vi "MFP assistant - Litho object manager.vi"(11 "Cluster":T1={"Objects to enable"=["r3", "p0", "p3"], "Only enable items in array ?"=FALSE, "All objects"=enum."Do nothing", "Funnel"=enum."Do nothing", "Path"=enum."Do nothing", "Rectangle"=enum."Do nothing"}) -> ()   [LabVIEW 2016]
uses:
  <userlib>/LevyLab/General AFM Lithography/subVIs/Global Variables.vi
panel:
  out "error out":errorcluster
  in  "error in (no error)":errorcluster
  # "Priority Level: Only enable items in array ? > All objects > Funnel, Path, Rectangle"
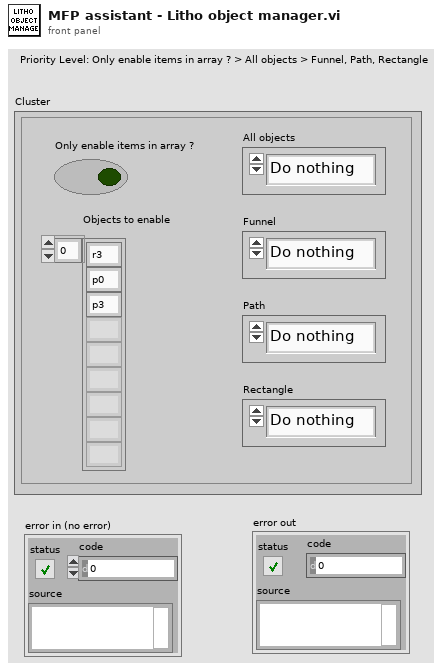
[diagram p1: front panel]
types:
  T1 = cluster{"Objects to enable":string[], "Only enable items in array ?":bool, "All objects":enum16{"Do nothing", "Disable all", "Enable all"}, "Funnel":enum16{"Do nothing", "Disable all", "Enable all"}, "Path":enum16{"Do nothing", "Disable all", "Enable all"}, "Rectangle":enum16{"Do nothing", "Disable all", "Enable all"}}
  T2 = enum16{"Do nothing", "Disable all", "Enable all"}
  T3 = typedef "Funnel Properties - cluster.ctl" = cluster{"Enabled":bool, "Direction":u16, "Smooth Segments":dbl, "Bottom Segs.":dbl, "Speed (um/s)":T4, "Voltage (V)":T4, "Set Resistance":T7}
  T4 = typedef "Voltage - cluster.ctl" = cluster{"Schedule":T5, "Value":dbl, "Start Value":dbl, "End Value":dbl, "Min Value":dbl, "Max Value":dbl, "Duty Cycle (%)":dbl, "Signal Type":T6, "Cycle Number":dbl, "Phase (degrees)":dbl, "formula":string, "formula length (nm)":dbl, "formula resolution (nm)":dbl}
  T5 = typedef "Schedule - enum.ctl" = enum16{"Constant", "Ramp", "Fn. Generator", "Formula"}
  T6 = typedef "Signal Type - enum.ctl" = enum16{"Sine Wave", "Triangle Wave", "Square Wave", "Sawtooth Wave"}
  T7 = typedef "Resistor--enum.ctl" = enum16{"open", "discharge tip", "0 ohms", "100k ohm", "10M ohm", "1G ohm"}
  T8 = typedef "Path Properties - cluster.ctl" = cluster{"Enabled":bool, "Direction":u16, "Fill Orientation":u16, "Smooth Segments":dbl, "Fill Spacing":dbl, "Speed (um/s)":T4, "Voltage (V)":T4, "Set Resistance":T7}
  T9 = typedef "Rectangle Properties - cluster.ctl" = cluster{"Enabled":bool, "Direction":u16, "Fill Orientation":u16, "Fill Spacing":dbl, "Speed (um/s)":T4, "Voltage (V)":T4, "Set Resistance":T7}
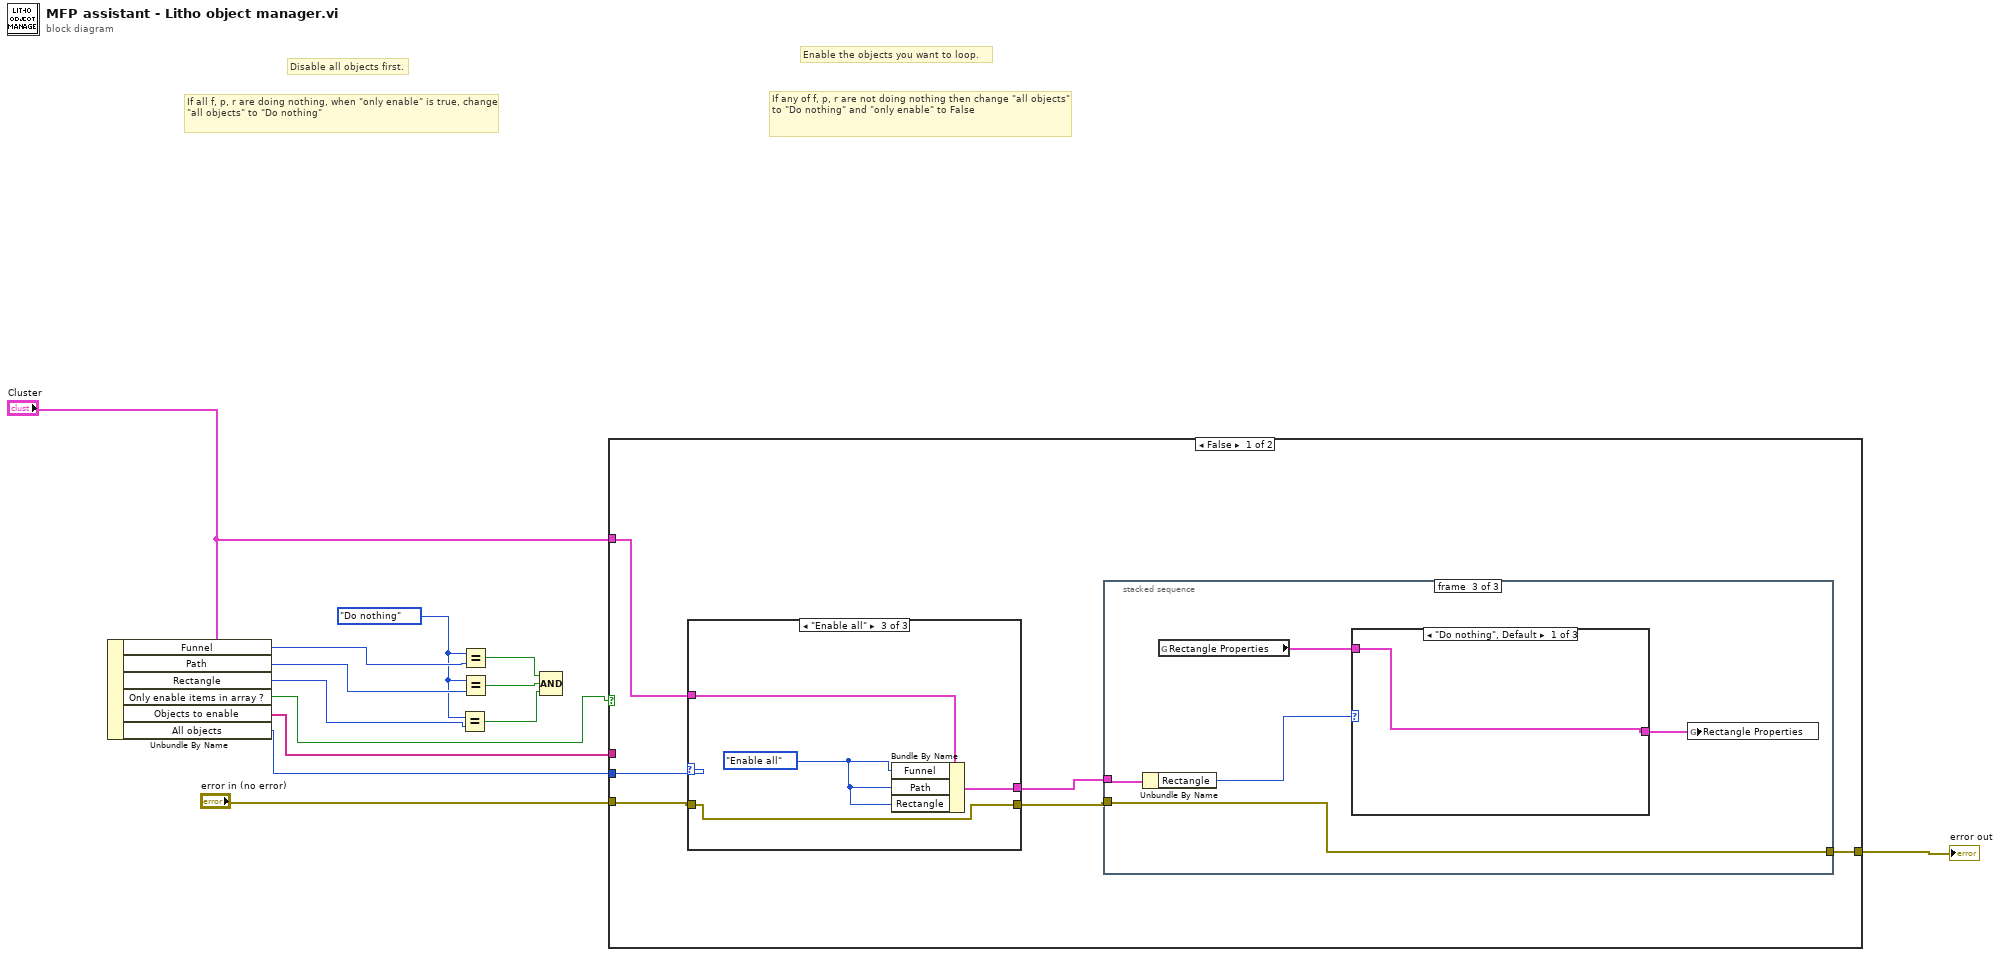
[diagram p0: block diagram]
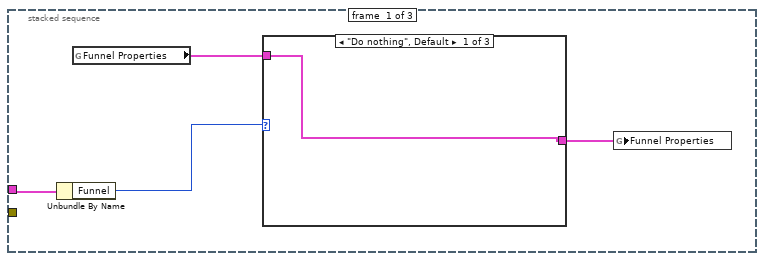
[diagram p2: hidden frame]
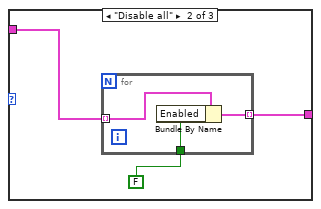
[diagram p3: hidden frame]
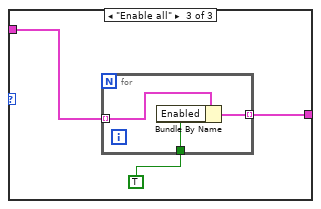
[diagram p4: hidden frame]
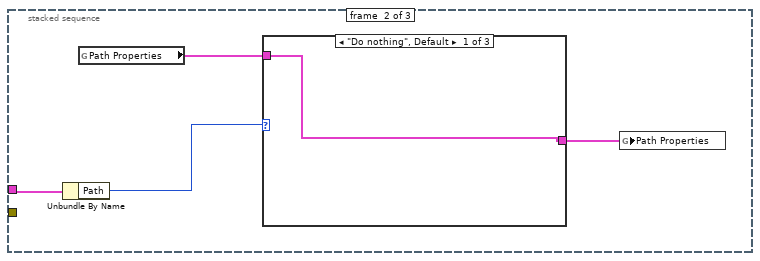
[diagram p5: hidden frame]
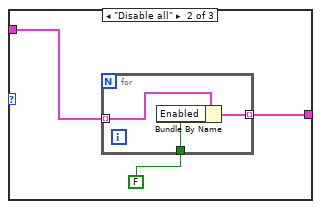
[diagram p6: hidden frame]
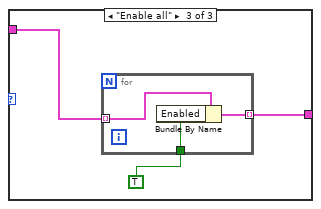
[diagram p7: hidden frame]
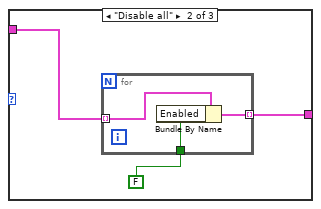
[diagram p8: hidden frame]
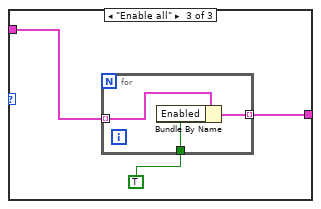
[diagram p9: hidden frame]
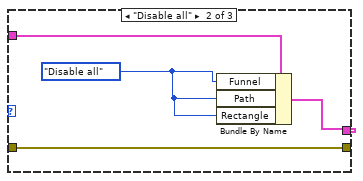
[diagram p11: hidden frame]
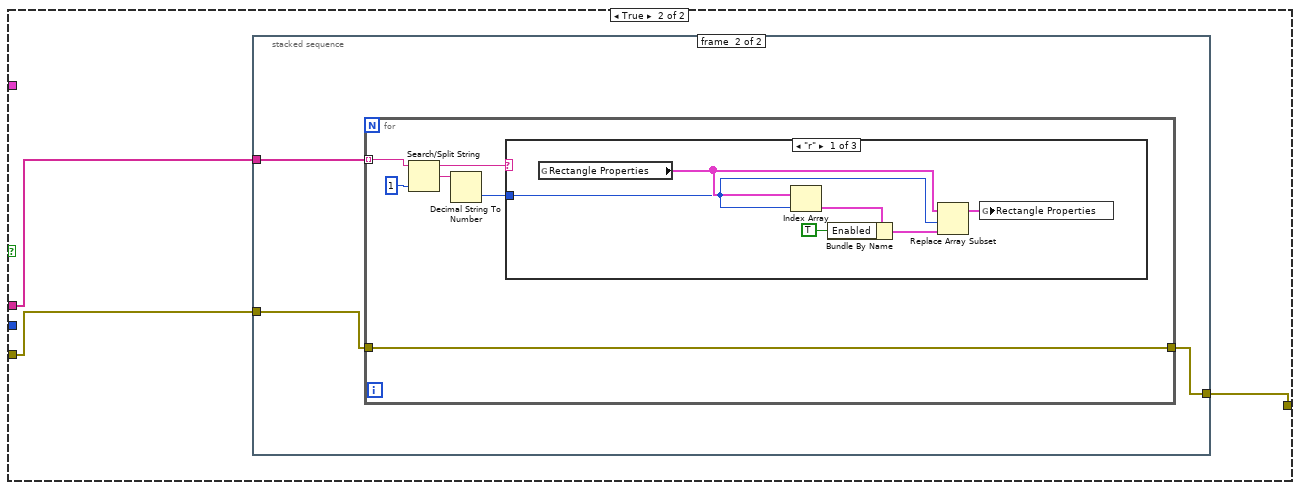
[diagram p12: hidden frame]
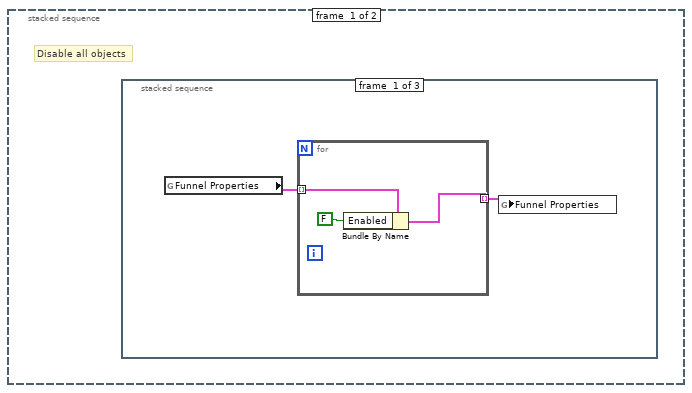
[diagram p13: hidden frame]
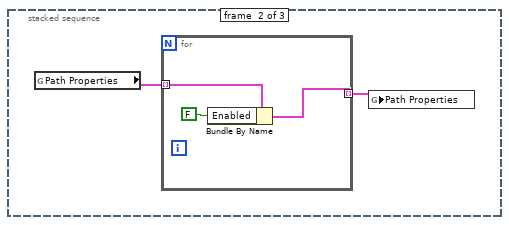
[diagram p14: hidden frame]
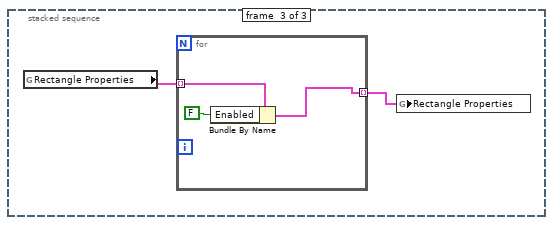
[diagram p15: hidden frame]
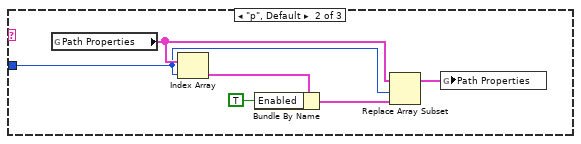
[diagram p16: hidden frame]
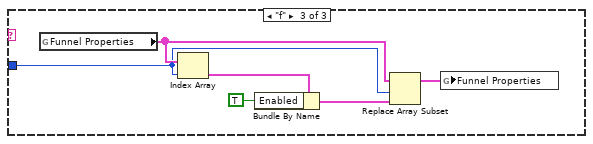
[diagram p17: hidden frame]
diagram:
  w11 = T2."Do nothing" ("Funnel")
  # "If any of f, p, r are not doing nothing then change \"all objects\" to \"Do nothing\" and \"only enable\" to False"
  # "If all f, p, r are doing nothing, when \"only enable\" is true, change \"all objects\" to \"Do nothing\""
  # "Disable all objects first."
  # "Enable the objects you want to loop."
  n1 = Unbundle By Name("Cluster") -> ("Funnel"=w13:T2, "Path"=w12:T2, "Rectangle"=w10:T2, "Only enable items in array ?"=w6:bool, "Objects to enable"=w5:string[], "All objects"=w3:T2)
  n2 = Equal?(x=w11, y=w10) -> (x = y?=w7:bool)
  n3 = Equal?(x=w11, y=w13) -> (x = y?=w9:bool)
  n4 = Equal?(x=w11, y=w12) -> (x = y?=w8:bool)
  n5 = Compound Arithmetic op=AND(w9, w8, w7) -> ()  [unwired: 1 out]
  n6 = case shown="False" w6 {
    tunnel: w5 -> [_ w84]
    tunnel: "error in (no error)" -> [w15 w83]
    tunnel: w3 -> [w19 _]
    tunnel: "Cluster" -> [w18 _]
    tunnel: [w16 w82] -> w1
    frame False {
      n7 = case shown="\"Enable all\"" w19 {
        tunnel: w18 -> [w72 w76 w80]
        tunnel: [w72 w74 w78] -> w17
        tunnel: w15 -> [w73 w75 w79]
        tunnel: [w73 w75 w79] -> w14
        frame "Do nothing", Default {
        }
        frame "Disable all" {
          w77 = T2."Disable all" ("Funnel")
          n8 = Bundle By Name(cluster=w76, "Funnel"=w77, "Path"=w77, "Rectangle"=w77) -> (w74:T1)
        }
        frame "Enable all" {
          w81 = T2."Enable all" ("Funnel")
          n9 = Bundle By Name(cluster=w80, "Funnel"=w81, "Path"=w81, "Rectangle"=w81) -> (w78:T1)
        }
      }
      n10 = stacked-sequence {
        tunnel: w17 -> [w21 w38 w56]
        tunnel: [_ _ w54] -> w16
        tunnel: w14 -> [_ _ w54]
        frame #0 {
          n11 = Unbundle By Name(w21) -> ("Funnel"=w20:T2)
          n12 = global read "Global Variables.vi" "Funnel Properties"() -> (w22:T3[])
          n13 = case shown="\"Do nothing\", Default" w20 {
            tunnel: [w24 w27 w33] -> w23
            tunnel: w22 -> [w24 w26 w32]
            frame "Do nothing", Default {
            }
            frame "Disable all" {
              n14 = for {
                tunnel: w26 -> [w30] mode=indexing
                tunnel: [w29] -> w27 mode=indexing
                tunnel: FALSE ("Enabled") -> [w28]
                n15 = Bundle By Name(cluster=w30, "Enabled"=w28) -> (w29:T3)
              }
            }
            frame "Enable all" {
              n16 = for {
                tunnel: w32 -> [w36] mode=indexing
                tunnel: [w35] -> w33 mode=indexing
                tunnel: TRUE ("Enabled") -> [w34]
                n17 = Bundle By Name(cluster=w36, "Enabled"=w34) -> (w35:T3)
              }
            }
          }
          n18 = global write "Global Variables.vi" "Funnel Properties"(w23) -> ()
        }
        frame #1 {
          n19 = Unbundle By Name(w38) -> ("Path"=w37:T2)
          n20 = global read "Global Variables.vi" "Path Properties"() -> (w39:T8[])
          n21 = case shown="\"Do nothing\", Default" w37 {
            tunnel: [w41 w44 w50] -> w40
            tunnel: w39 -> [w41 w43 w49]
            frame "Do nothing", Default {
            }
            frame "Disable all" {
              n22 = for {
                tunnel: w43 -> [w47] mode=indexing
                tunnel: [w46] -> w44 mode=indexing
                tunnel: FALSE ("Enabled") -> [w45]
                n23 = Bundle By Name(cluster=w47, "Enabled"=w45) -> (w46:T8)
              }
            }
            frame "Enable all" {
              n24 = for {
                tunnel: w49 -> [w53] mode=indexing
                tunnel: [w52] -> w50 mode=indexing
                tunnel: TRUE ("Enabled") -> [w51]
                n25 = Bundle By Name(cluster=w53, "Enabled"=w51) -> (w52:T8)
              }
            }
          }
          n26 = global write "Global Variables.vi" "Path Properties"(w40) -> ()
        }
        frame #2 {
          n27 = Unbundle By Name(w56) -> ("Rectangle"=w55:T2)
          n28 = global read "Global Variables.vi" "Rectangle Properties"() -> (w57:T9[])
          n29 = case shown="\"Do nothing\", Default" w55 {
            tunnel: [w59 w62 w68] -> w58
            tunnel: w57 -> [w59 w61 w67]
            frame "Do nothing", Default {
            }
            frame "Disable all" {
              n30 = for {
                tunnel: w61 -> [w65] mode=indexing
                tunnel: [w64] -> w62 mode=indexing
                tunnel: FALSE ("Enabled") -> [w63]
                n31 = Bundle By Name(cluster=w65, "Enabled"=w63) -> (w64:T9)
              }
            }
            frame "Enable all" {
              n32 = for {
                tunnel: w67 -> [w71] mode=indexing
                tunnel: [w70] -> w68 mode=indexing
                tunnel: TRUE ("Enabled") -> [w69]
                n33 = Bundle By Name(cluster=w71, "Enabled"=w69) -> (w70:T9)
              }
            }
          }
          n34 = global write "Global Variables.vi" "Rectangle Properties"(w58) -> ()
        }
      }
    }
    frame True {
      n35 = stacked-sequence {
        tunnel: w84 -> [_ w102]
        tunnel: w83 -> [_ w101]
        tunnel: [_ w100] -> w82
        frame #0 {
          # "Disable all objects"
          n36 = stacked-sequence {
            frame #0 {
              n37 = global read "Global Variables.vi" "Funnel Properties"() -> (w85:T3[])
              n38 = for {
                tunnel: w85 -> [w88] mode=indexing
                tunnel: [w87] -> w86 mode=indexing
                n39 = Bundle By Name(cluster=w88, "Enabled"=FALSE) -> (w87:T3)
              }
              n40 = global write "Global Variables.vi" "Funnel Properties"(w86) -> ()
            }
            frame #1 {
              n41 = global read "Global Variables.vi" "Path Properties"() -> (w90:T8[])
              n42 = for {
                tunnel: w90 -> [w93] mode=indexing
                tunnel: [w92] -> w91 mode=indexing
                n43 = Bundle By Name(cluster=w93, "Enabled"=FALSE) -> (w92:T8)
              }
              n44 = global write "Global Variables.vi" "Path Properties"(w91) -> ()
            }
            frame #2 {
              n45 = global read "Global Variables.vi" "Rectangle Properties"() -> (w95:T9[])
              n46 = for {
                tunnel: w95 -> [w98] mode=indexing
                tunnel: [w97] -> w96 mode=indexing
                n47 = Bundle By Name(cluster=w98, "Enabled"=FALSE) -> (w97:T9)
              }
              n48 = global write "Global Variables.vi" "Rectangle Properties"(w96) -> ()
            }
          }
        }
        frame #1 {
          n49 = for {
            tunnel: w102 -> [w104] mode=indexing
            tunnel: [w103] -> w100
            tunnel: w101 -> [w103]
            n50 = Search/Split String(string=w104, offset (0)=1) -> (substring before match=w106:string, match + rest of string=w107:string)  [unwired: 1 in, 1 out]
            n51 = Decimal String To Number(string=w107) -> (number=w105:i32)  [unwired: 2 in, 1 out]
            n52 = case shown="\"r\"" w106 {
              tunnel: w105 -> [w109 w115 w121]
              frame "r" {
                n53 = global read "Global Variables.vi" "Rectangle Properties"() -> (w113:T9[])
                n54 = Index Array(array=w113, index=w109) -> (element=w110:T9)
                n55 = Bundle By Name(cluster=w110, "Enabled"=TRUE) -> (w111:T9)
                n56 = Replace Array Subset(array=w113, new element=w111, index=w109) -> (w114:T9[])
                n57 = global write "Global Variables.vi" "Rectangle Properties"(w114) -> ()
              }
              frame "p", Default {
                n58 = global read "Global Variables.vi" "Path Properties"() -> (w119:T8[])
                n59 = Index Array(array=w119, index=w115) -> (element=w116:T8)
                n60 = Bundle By Name(cluster=w116, "Enabled"=TRUE) -> (w117:T8)
                n61 = Replace Array Subset(array=w119, new element=w117, index=w115) -> (w120:T8[])
                n62 = global write "Global Variables.vi" "Path Properties"(w120) -> ()
              }
              frame "f" {
                n63 = global read "Global Variables.vi" "Funnel Properties"() -> (w125:T3[])
                n64 = Index Array(array=w125, index=w121) -> (element=w122:T3)
                n65 = Bundle By Name(cluster=w122, "Enabled"=TRUE) -> (w123:T3)
                n66 = Replace Array Subset(array=w125, new element=w123, index=w121) -> (w126:T3[])
                n67 = global write "Global Variables.vi" "Funnel Properties"(w126) -> ()
              }
            }
          }
        }
      }
    }
  }
  "error out" <- w1
